vi "Stop Core.vi"(10 "final error code":i32, 11 "HamaCam in":refnum<class "HamaCam.lvclass">) -> (3 "HamaCam out":refnum<class "HamaCam.lvclass">)   [LabVIEW 2023, in "HamaCam.lvlib" / "HamaCam.lvclass"]
doc: "(<B>Filename</B>: Actor Framework.lvlib:Actor.lvclass:Stop Core.vi)\n\nDefines what the actor does before it stops. Use the <B>final error code</B> input to determine whether the actor shut down in response to an error.\n\nBy default, this method passes the Stop message along to all auto-stop nested actors. A descendant class may override this method to define additional behavior, such as shutting down any processes the actor initiated in its override of the Actor Core method."
uses:
  HamaCam.lvclass
  <vilib>/ActorFramework/Actor/Actor.lvclass
  HamaCam.lvclass/HamaCam.ctl
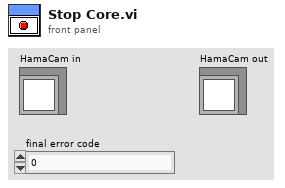
[diagram p1: front panel]
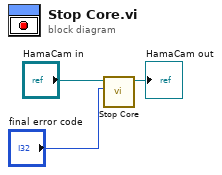
[diagram p0: block diagram]
diagram:
  n1 = call-parent "Stop Core.vi"("final error code"="final error code", "Actor in"="HamaCam in") -> ("Actor out"=→"HamaCam out":refnum<class "HamaCam.lvclass">)  [unwired: 9 in]
